vi "LIN Errors Error.vi"(11 "Errors":T1) -> (3 "Error":bool)   [LabVIEW 2020, in "Linearisierung v2.lvlib" / "SpanEinstellungen.lvlib"]
uses:
  SpanEinstellungen.lvlib
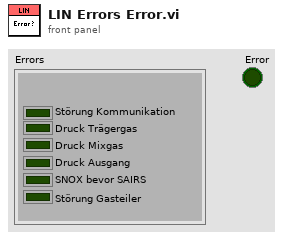
[diagram p1: front panel]
types:
  T1 = cluster{"Störung Kommunikation":bool, "Pressure carrier gas":bool, "Pressure diluted gas":bool, "Outlet Pressure":bool, "SNOX before SAIR":bool, "Störung Gasteiler":bool}
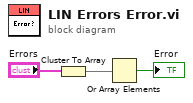
[diagram p0: block diagram]
diagram:
  n1 = Cluster To Array(cluster="Errors") -> (array=w2:bool[])
  n2 = Or Array Elements(Boolean array=w2) -> (logical OR=→"Error":bool)
